vi "Find length or distance.vi"() -> ()   [LabVIEW 2015]
uses:
  <vilib>/vision/NI_Vision_Development_Module.lvlib
panel:
  out "Image":T1(plugin-control)
  out "Length or Distance (pixels)":sgl
  in  "Image to View":path
  in  "stop":bool
  # "INSTRUCTIONS:\n1) Select an Image to View\n2) Run the VI\n3) Select an ROI tool at the left of\n     the image display\n4) Click and drag to draw a line if\n    you selected the line tool, or\n    Ctrl+click to select two points \n    if you selected the point tool\n5) The VI will calculate the length\n    of the line or the distance\n    between the two points"
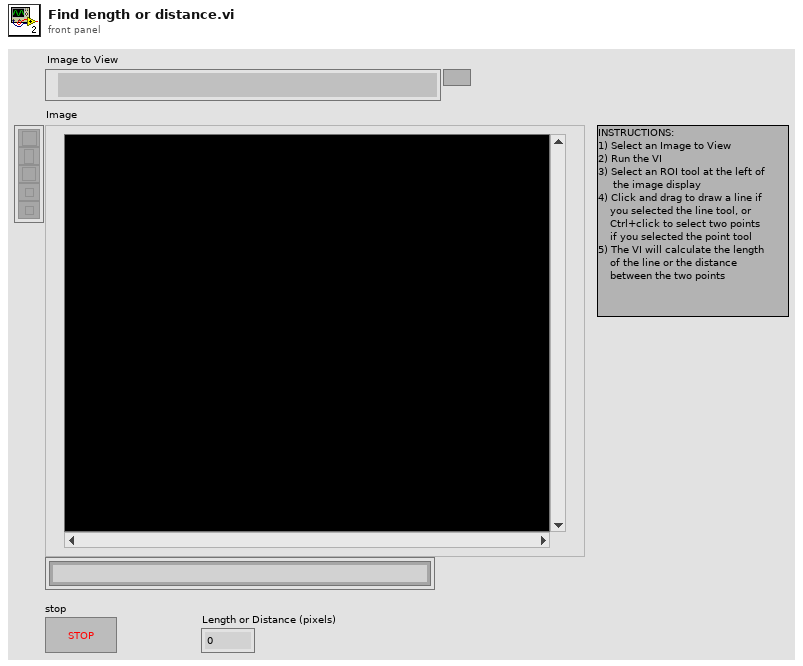
[diagram p1: front panel]
types:
  T1 = typedef "IMAQ Image.ctl" = refnum<image>
  T2 = cluster{"Global Rectangle":i32[], "Contours":cluster{"Contour Type":u32, "ROI Type":u32, "Points":i32[]}[]}
  T3 = typedef "ROI Descriptor" = cluster{"Global Rectangle":i32[], "Contours":cluster{"ID":enum32{"External", "Internal"}, "Type":u32, "Coordinates":i32[]}[]}
  T4 = typedef "IMAQ Point" = cluster{"X":sgl, "Y":sgl}
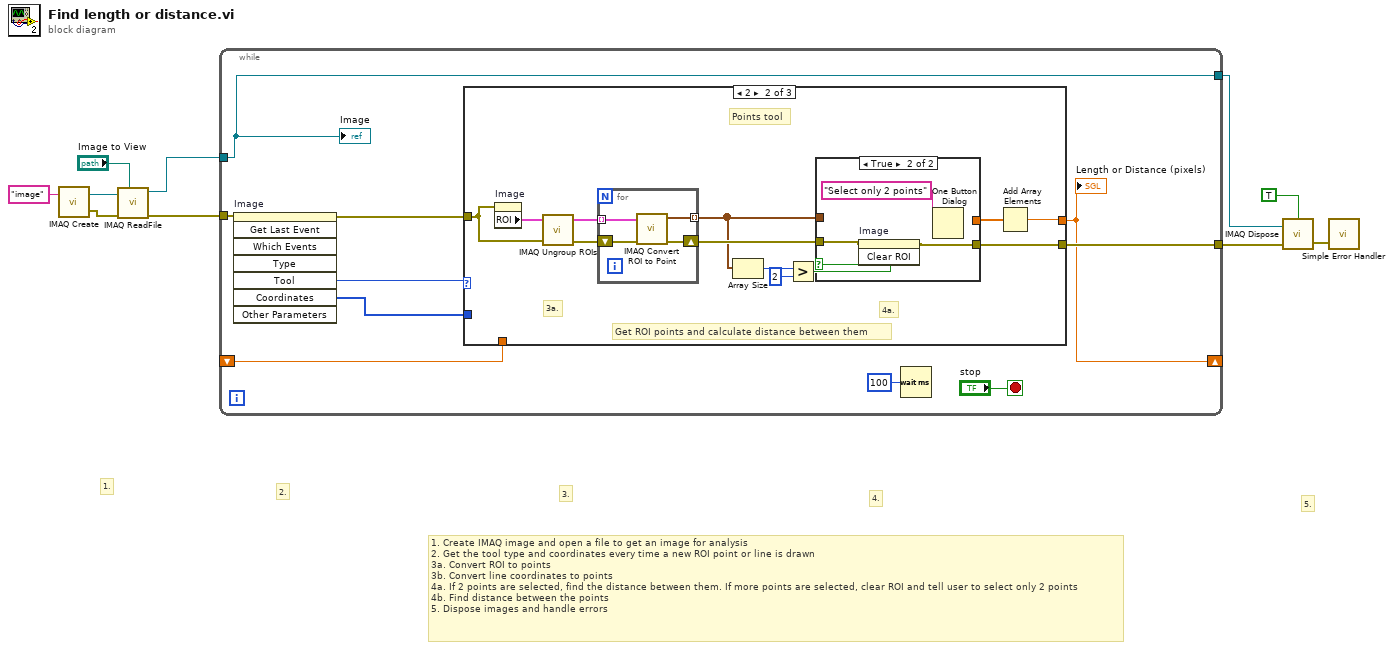
[diagram p0: block diagram]
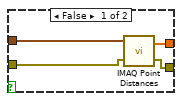
[diagram p3: hidden frame]
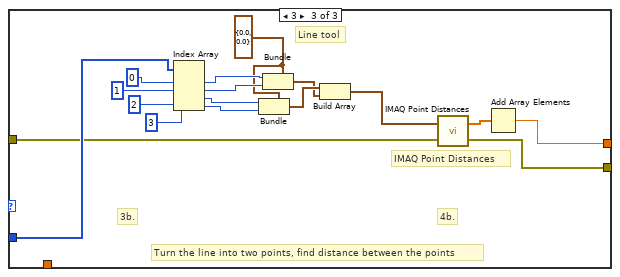
[diagram p4: hidden frame]
diagram:
  # "5."
  # "1. Create IMAQ image and open a file to get an image for analysis\n2. Get the tool type and coordinates every time a new ROI point or line is drawn\n3a. Convert ROI to points\n3b. Convert line coordinates to points\n4a. If 2 points are selected, find the distance between them. If more points are selected, clear ROI and tell user to select only 2 points\n4b. Find distance between the points\n5. Dispose images and handle errors"
  # "4."
  # "3."
  # "2."
  # "1."
  n1 = call "IMAQ Create"("Image Name"="image") -> ("New Image"=w9:T1, "error out"=w10:errorcluster)  [unwired: 4 in]
  n2 = call "IMAQ ReadFile"("File Path"="Image to View", "error in (no error)"=w10, "Image"=w9) -> ("error out"=w7:errorcluster, "Image Out"=w8:T1)  [unwired: 4 in, 3 out]
  n3 = while {
    tunnel: w8 -> [w11]
    tunnel: [w20] -> w3
    tunnel: w7 -> [w14]
    shift-right: [w17] -> _
    shift-left: _ -> [w16]
    tunnel: [w11] -> w4
    stop <- "stop" stop-if-true
    n4 = invoke on="Image" class="ImageControl" method="Get Last Event"(error in=w14) -> (error out=w15:errorcluster, "Tool"=w13:i32, "Coordinates"=w12:i32[])  [unwired: 7 in, 5 out]
    n5 = case shown="2" w13 {
      tunnel: w12 -> [_ _ w51]
      tunnel: [w22 w27 w47] -> w20
      tunnel: [w21 w25 w48] -> w17
      tunnel: w15 -> [w22 w24 w46]
      tunnel: w16 -> [w21 _ _]
      frame 0, Default {
        # "Do nothing if no new ROI is selected"
      }
      frame 2 {
        # "Points tool"
        # "4a."
        # "3a."
        # "Get ROI points and calculate distance between them"
        n6 = property on="Image" class="ImageControl"(error in=w24) -> ("ROI"=w23:T2)  [unwired: 1 in, 2 out]
        n7 = call "IMAQ Ungroup ROIs"("error in (no error)"=w24, "ROI Descriptor"=w23) -> ("error out"=w34:errorcluster, "ROI Descriptors out"=w33:T3[])  [unwired: 2 out]
        n8 = for {
          shift-right: [w42] -> w32
          shift-left: w34 -> [w45]
          tunnel: w33 -> [w44] mode=indexing
          tunnel: [w43] -> w31 mode=indexing
          n9 = call "IMAQ Convert ROI to Point"("error in (no error)"=w45, "ROI Descriptor"=w44) -> ("error out"=w42:errorcluster, "Point"=w43:T4)  [unwired: 7 out]
        }
        n10 = Array Size(array=w31) -> (size(s)=w30:i32)
        n11 = Greater?(x=w30, y=2) -> (0:w28:bool)
        n12 = case shown="True" w28 {
          tunnel: w32 -> [w38 w40]
          tunnel: w31 -> [w37 _]
          tunnel: [w36 w39] -> w27
          tunnel: [w35 _] -> w26
          frame False {
            n13 = call "IMAQ Point Distances"("Points"=w37, "error in (no error)"=w38) -> ("Distances"=w35:sgl[], "error out"=w36:errorcluster)  [unwired: 3 in]
          }
          frame True {
            n14 = invoke on="Image" class="ImageControl" method="Clear ROI"(error in=w40) -> (error out=w39:errorcluster)  [unwired: 2 in, 2 out]
            n15 = One Button Dialog(message="Select only 2 points") -> ()  [unwired: 1 in, 1 out]
          }
        }
        n16 = Add Array Elements(numeric array=w26) -> (sum=w25:sgl)
      }
      frame 3 {
        w50 = cluster{"X":sgl, "Y":sgl} {"X"=0.0, "Y"=0.0}
        # "Line tool"
        # "4b."
        # "3b."
        # "Turn the line into two points, find distance between the points"
        # "IMAQ Point Distances"
        n17 = Index Array(array=w51, index #1=0 ("index"), index #2=1 ("index"), index #3=2 ("index"), index #4=3 ("index")) -> (element #1=w58:i32, element #2=w57:i32, element #3=w56:i32, element #4=w55:i32)
        n18 = Bundle(cluster=w50, "X"=w56, "Y"=w55) -> (w54:cluster{"X":sgl, "Y":sgl})
        n19 = Bundle(cluster=w50, "X"=w58, "Y"=w57) -> (w53:cluster{"X":sgl, "Y":sgl})
        n20 = Build Array(w54, w53) -> (w52:cluster{"X":sgl, "Y":sgl}[])
        n21 = call "IMAQ Point Distances"("Points"=w52, "error in (no error)"=w46) -> ("Distances"=w49:sgl[], "error out"=w47:errorcluster)  [unwired: 3 in]
        n22 = Add Array Elements(numeric array=w49) -> (sum=w48:sgl)
      }
    }
    "Length or Distance (pixels)" <- w17
    n23 = Wait (ms)(milliseconds to wait=u32 100) -> ()  [unwired: 1 out]
    "Image" <- w11
  }
  n24 = call "IMAQ Dispose"("All Images? (No)"=TRUE, "Image"=w4, "error in (no error)"=w3) -> ("error out"=w1:errorcluster)  [unwired: 3 in]
  n25 = call <vilib>:"Simple Error Handler.vi"("error in (no error)"=w1) -> ()  [unwired: 4 in, 5 out]
